vi "subVI_explodeArray.vi"(7 "Array":variant[](array[variant])) -> (6 "x":variant, 8 "y":variant, 10 "z":variant)   [LabVIEW 2010]
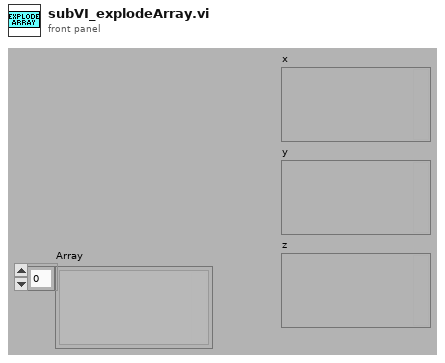
[diagram p1: front panel]
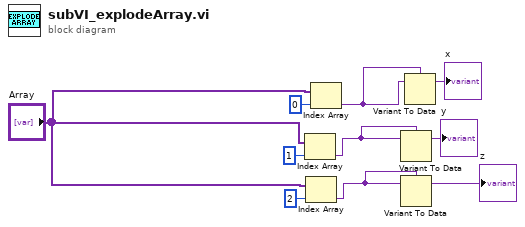
[diagram p0: block diagram]
diagram:
  n1 = Index Array(array="Array", index=1) -> (element=w5:variant)
  n2 = Index Array(array="Array", index=2) -> (element=w4:variant)
  n3 = Index Array(array="Array", index=0) -> (element=w6:variant)
  n4 = Variant To Data(Variant=w5, type=w5) -> (data=→"y":variant)  [unwired: 1 in, 1 out]
  n5 = Variant To Data(Variant=w4, type=w4) -> (data=→"z":variant)  [unwired: 1 in, 1 out]
  n6 = Variant To Data(Variant=w6, type=w6) -> (data=→"x":variant)  [unwired: 1 in, 1 out]
